vi "CalculatePhaseMagnitude_5761.vi"(8 "unwrap phase":bool, 9 "phase reference channel":i32, 10 "previous phase":dbl[](array[numeric]), 11 "data":dbl[][](array[numeric])) -> (1 "last phase":dbl[](array[numeric]), 2 "Magnitude":dbl[][](array[numeric]), 3 "Phase":dbl[][](array[numeric]))   [LabVIEW 2013]
uses:
  <vilib>/Analysis/coordinate.llb/Angle Units.ctl
  <vilib>/Analysis/NI_AALPro.lvlib
  <vilib>/Analysis/NI_AAL_Angle.lvlib
panel:
  # "each row is I and then Q of one channel"
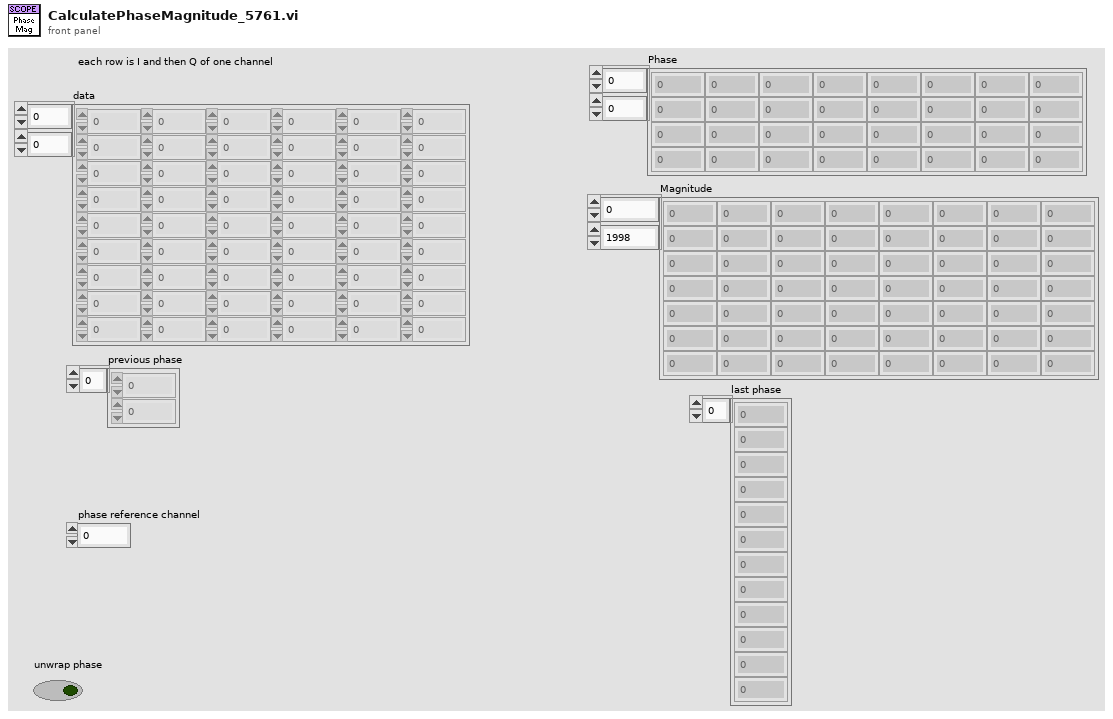
[diagram p1: front panel]
types:
  T1 = typedef "NI_AAL_Angle.lvlib/Angle Units.ctl" = i32
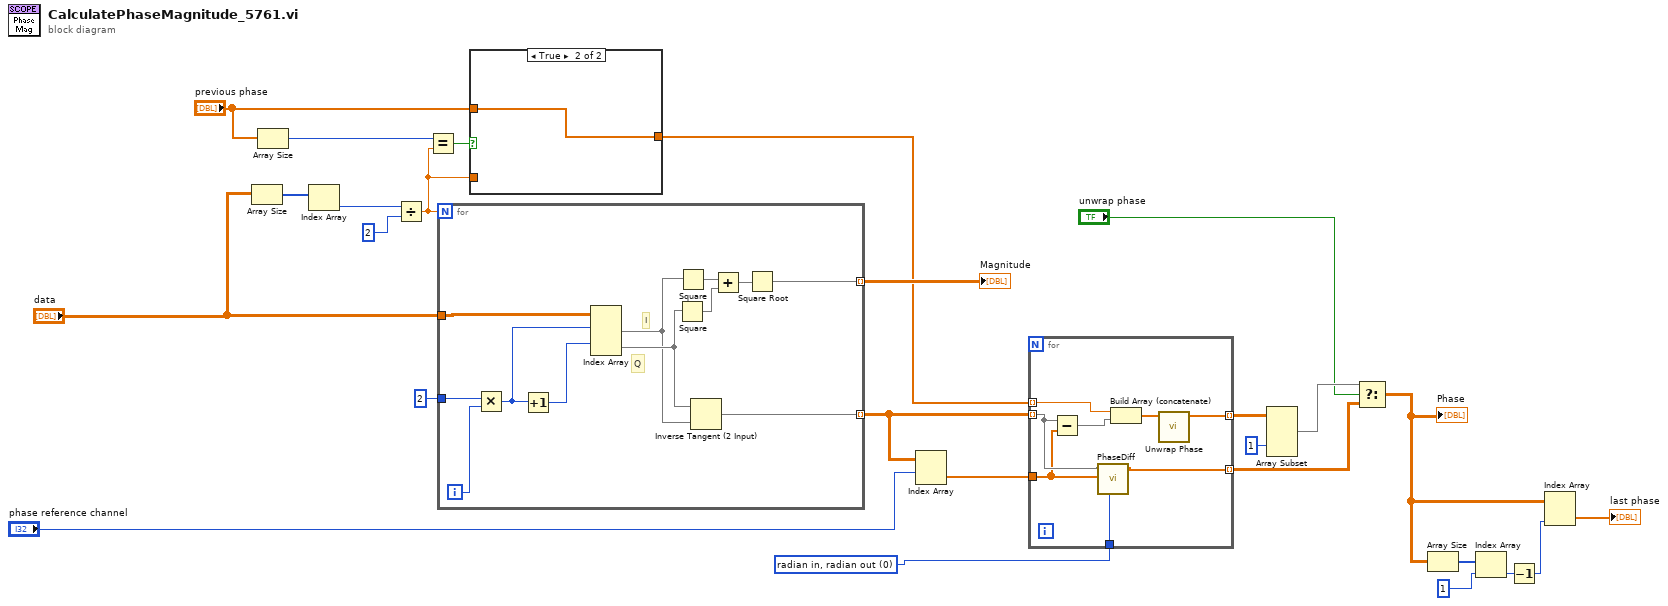
[diagram p0: block diagram]
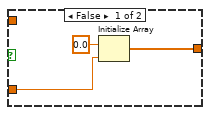
[diagram p2: hidden frame]
diagram:
  w11 = T1 0 items=["radian in, radian out", "radian in, degree out", "degree in, degree out", "degree in, radian out"] ("angle units")
  n1 = Array Size(array="data") -> (size(s)=w17:i32[])
  n2 = Array Size(array="previous phase") -> (size(s)=w9:i32)
  n3 = Index Array(array=w17) -> (element=w16:i32)  [unwired: 1 in]
  n4 = Divide(x=w16, y=2) -> (x/y=w6:dbl)
  n5 = Equal?(x=w9, y=w6) -> (x = y?=w8:bool)
  n6 = for {
    N: w6 -> [_]
    tunnel: "data" -> [w38]
    tunnel: 2 ("y") -> [w37]
    tunnel: [w28] -> w25 mode=indexing
    tunnel: [w27] -> w10 mode=indexing
    i -> [w34]
    # "Q"
    # "I"
    n7 = Multiply(x=w37, y=w34) -> (x*y=w36:i32)
    n8 = Increment(x=w36) -> (x+1=w35:i32)
    n9 = Index Array(array=w38, index (row) #1=w36, index (row) #2=w35) -> (element #1=w29:dbl[], element #2=w30:dbl[])  [unwired: 2 in]
    n10 = Square(x=w30) -> (x^2=w32:dbl[])
    n11 = Square(x=w29) -> (x^2=w33:dbl[])
    n12 = Inverse Tangent (2 Input)(1:w29, 2:w30) -> (0:w27:dbl[])
    n13 = Add(x=w33, y=w32) -> (x+y=w31:dbl[])
    n14 = Square Root(x=w31) -> (sqrt(x)=w28:dbl[])
  }
  "Magnitude" <- w25
  n15 = case shown="True" w8 {
    tunnel: "previous phase" -> [_ w42]
    tunnel: [w39 w42] -> w5
    tunnel: w6 -> [w40 _]
    frame False {
      n16 = Initialize Array(0.0 ("element"), w40) -> (w39:dbl[])
    }
    frame True {
    }
  }
  n17 = Index Array(array=w10, index (row)="phase reference channel") -> (element=w18:dbl[])  [unwired: 1 in]
  n18 = for {
    tunnel: w10 -> [w46] mode=indexing
    tunnel: w18 -> [w45]
    tunnel: [w50] -> w12 mode=indexing
    tunnel: w5 -> [w49] mode=indexing
    tunnel: [w44] -> w2 mode=indexing
    tunnel: w11 -> [w43]
    n19 = Subtract(x=w46, y=w45) -> (x-y=w47:dbl[])
    n20 = call "PhaseDiff.vi"("angle units"=w43, "Angle 2"=w45, "Angle 1"=w46) -> ("Absolute Angle Difference"=w44:dbl[])  [unwired: 5 in]
    n21 = Build Array (concatenate)(w49, w47) -> (w48:dbl[])
    n22 = call <vilib>:"Unwrap Phase.vi"("Phase"=w48) -> ("Unwrapped Phase"=w50:dbl[])  [unwired: 9 in, 1 out]
  }
  n23 = Array Subset(array=w12, index (col)=1 ("index")) -> (w4:dbl[][])  [unwired: 3 in]
  n24 = Select(t=w4, s="unwrap phase", f=w2) -> (s? t:f=w3:dbl[][])
  "Phase" <- w3
  n25 = Array Size(array=w3) -> (size(s)=w23:i32[])
  n26 = Index Array(array=w23, index=1) -> (element=w22:i32)
  n27 = Decrement(x=w22) -> (x-1=w20:i32)
  n28 = Index Array(array=w3, index (col)=w20) -> (element=→"last phase":dbl[])  [unwired: 1 in]
